vi "Benchmark Replace.vi"() -> ()   [LabVIEW 2017]
uses:
  Source/LookupTable/LookupTable.lvclass/LookupTable.ctl
  fb17a209-de8c-4f41-abf7-ab837125ba6b.vi
  bfc32706-22d1-41c7-b150-1593975a2be3.vi
  Source/LookupTable/Read Table Reference.vi
  Source/LookupTable/LookupTable.lvclass
panel:
  in  "Numeric":i32=100000
  out "Waveform Chart":cluster{dbl, dbl, dbl}(graph)
  out "Variant DVR":dbl
  out "Variant by value":dbl
  out "Composed Lookup Table":dbl
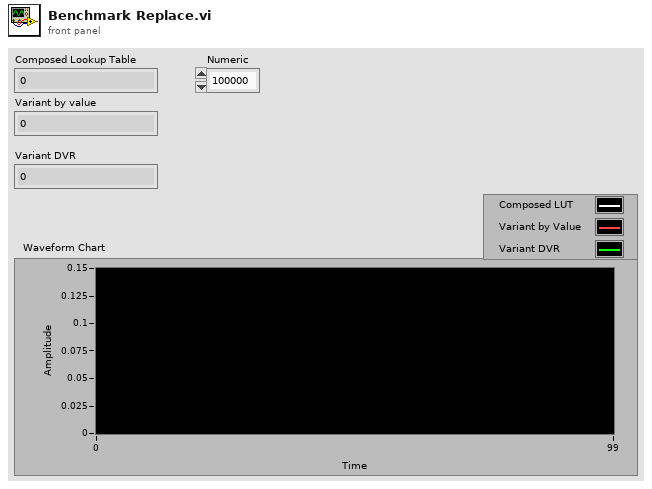
[diagram p1: front panel]
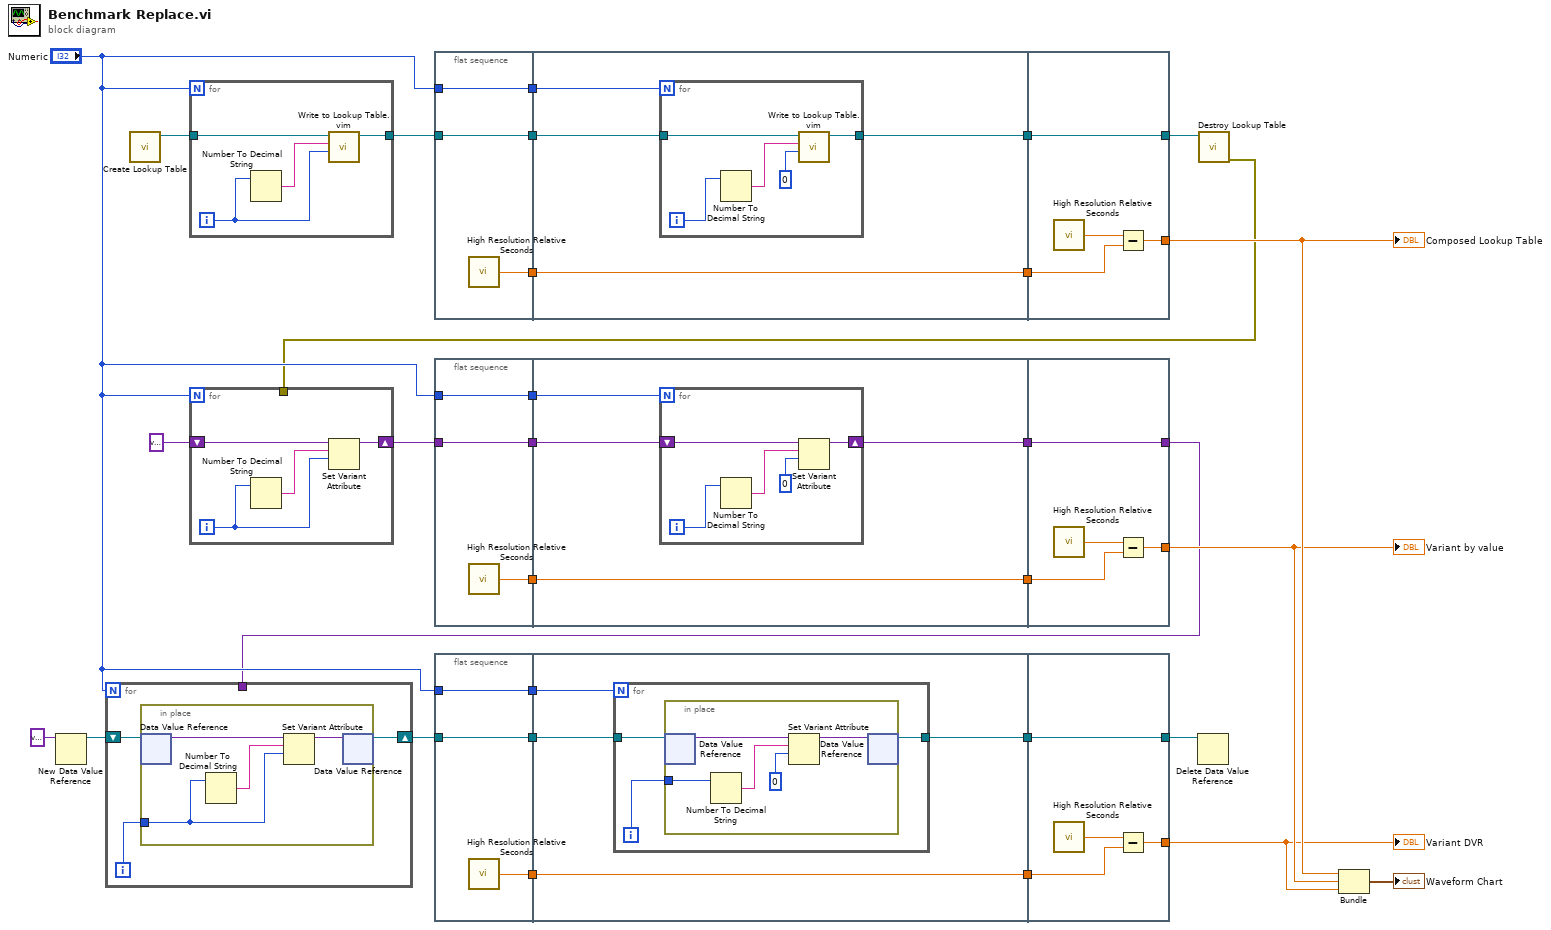
[diagram p0: block diagram]
diagram:
  n1 = New Data Value Reference(data value=variant) -> (data value reference=w11:refnum<data-value>)  [unwired: 1 in, 1 out]
  n2 = for {
    N: "Numeric" -> [_]
    shift-right: [w33] -> w10
    shift-left: w11 -> [w34]
    tunnel: w2 -> [_]
    i -> [w32]
    n3 = in-place {
      in-place-border: w32 -> [w35]
      n4 = in-place-dvr #1(w34) -> (w37:variant)  [unwired: 1 out]
      n5 = Number To Decimal String(number=w35) -> (decimal integer string=w38:string)  [unwired: 1 in]
      n6 = Set Variant Attribute(Variant=w37, name=w38, value=w35) -> (Variant out=w36:variant)  [unwired: 1 in, 2 out]
      n7 = in-place-dvr #1(w36) -> (w33:refnum<data-value>)  [unwired: 1 out]
    }
  }
  n8 = call "Create Lookup Table.vi"() -> ("LookupTable Reference"=w26:refnum<data-value>)  [unwired: 10 in, 1 out]
  n9 = for {
    N: "Numeric" -> [_]
    tunnel: [w40] -> w24
    tunnel: w26 -> [w39]
    i -> [w41]
    n10 = Number To Decimal String(number=w41) -> (decimal integer string=w42:string)  [unwired: 1 in]
    n11 = call "Write to Lookup Table.vim"("Item"=w41, "Item Name"=w42, "LookupTable Reference"=w39) -> ("LookupTable Reference Out"=w40:refnum<data-value>)  [unwired: 6 in, 2 out]
  }
  n12 = flat-sequence {
    tunnel: [w45] -> w31
    tunnel: [w44] -> w25
    tunnel: w24 -> [w44]
    tunnel: [w43] -> w19
    tunnel: "Numeric" -> [w43]
    tunnel: w31 -> [w49]
    tunnel: [w49] -> w30
    tunnel: w25 -> [w48]
    tunnel: [w47] -> w22
    tunnel: w19 -> [w46]
    tunnel: w30 -> [w57]
    tunnel: [w56] -> w7
    tunnel: [w55] -> w23
    tunnel: w22 -> [w55]
    frame #0 {
      n13 = call <vilib>:"High Resolution Relative Seconds.vi"() -> ("relative seconds"=w45:dbl)
    }
    frame #1 {
      n14 = for {
        N: w46 -> [_]
        tunnel: [w52] -> w47
        tunnel: w48 -> [w51]
        i -> [w53]
        n15 = Number To Decimal String(number=w53) -> (decimal integer string=w54:string)  [unwired: 1 in]
        n16 = call "Write to Lookup Table.vim"("Item"=0, "Item Name"=w54, "LookupTable Reference"=w51) -> ("LookupTable Reference Out"=w52:refnum<data-value>)  [unwired: 6 in, 2 out]
      }
    }
    frame #2 {
      n17 = call <vilib>:"High Resolution Relative Seconds.vi"() -> ("relative seconds"=w58:dbl)
      n18 = Subtract(x=w58, y=w57) -> (x-y=w56:dbl)
    }
  }
  n19 = flat-sequence {
    tunnel: [w61] -> w29
    tunnel: [w60] -> w21
    tunnel: w20 -> [w60]
    tunnel: "Numeric" -> [w59]
    tunnel: [w59] -> w18
    tunnel: w29 -> [w65]
    tunnel: [w65] -> w28
    tunnel: w21 -> [w64]
    tunnel: w18 -> [w63]
    tunnel: [w62] -> w1
    tunnel: w28 -> [w73]
    tunnel: [w72] -> w6
    tunnel: [w71] -> w2
    tunnel: w1 -> [w71]
    frame #0 {
      n20 = call <vilib>:"High Resolution Relative Seconds.vi"() -> ("relative seconds"=w61:dbl)
    }
    frame #1 {
      n21 = for {
        N: w63 -> [_]
        shift-right: [w70] -> w62
        shift-left: w64 -> [w67]
        i -> [w68]
        n22 = Number To Decimal String(number=w68) -> (decimal integer string=w69:string)  [unwired: 1 in]
        n23 = Set Variant Attribute(Variant=w67, name=w69, value=0) -> (Variant out=w70:variant)  [unwired: 1 in, 2 out]
      }
    }
    frame #2 {
      n24 = call <vilib>:"High Resolution Relative Seconds.vi"() -> ("relative seconds"=w74:dbl)
      n25 = Subtract(x=w74, y=w73) -> (x-y=w72:dbl)
    }
  }
  n26 = flat-sequence {
    tunnel: [w77] -> w17
    tunnel: [w76] -> w16
    tunnel: w10 -> [w76]
    tunnel: "Numeric" -> [w75]
    tunnel: [w75] -> w15
    tunnel: w17 -> [w81]
    tunnel: [w81] -> w14
    tunnel: w16 -> [w80]
    tunnel: w15 -> [w78]
    tunnel: [w79] -> w13
    tunnel: w14 -> [w92]
    tunnel: [w91] -> w5
    tunnel: [w90] -> w9
    tunnel: w13 -> [w90]
    frame #0 {
      n27 = call <vilib>:"High Resolution Relative Seconds.vi"() -> ("relative seconds"=w77:dbl)
    }
    frame #1 {
      n28 = for {
        N: w78 -> [_]
        tunnel: [w83] -> w79
        tunnel: w80 -> [w82]
        i -> [w84]
        n29 = in-place {
          in-place-border: w84 -> [w88]
          n30 = in-place-dvr #2(w82) -> (w87:variant)  [unwired: 1 out]
          n31 = Number To Decimal String(number=w88) -> (decimal integer string=w89:string)  [unwired: 1 in]
          n32 = Set Variant Attribute(Variant=w87, name=w89, value=0) -> (Variant out=w86:variant)  [unwired: 1 in, 2 out]
          n33 = in-place-dvr #2(w86) -> (w83:refnum<data-value>)  [unwired: 1 out]
        }
      }
    }
    frame #2 {
      n34 = call <vilib>:"High Resolution Relative Seconds.vi"() -> ("relative seconds"=w93:dbl)
      n35 = Subtract(x=w93, y=w92) -> (x-y=w91:dbl)
    }
  }
  n36 = Delete Data Value Reference(data value reference=w9) -> ()  [unwired: 1 in, 2 out]
  n37 = call "Destroy Lookup Table.vi"("LookupTable Reference"=w23) -> ("error out"=w3:errorcluster)  [unwired: 10 in]
  n38 = for {
    N: "Numeric" -> [_]
    shift-right: [w97] -> w20
    shift-left: variant -> [w94]
    tunnel: w3 -> [_]
    i -> [w95]
    n39 = Number To Decimal String(number=w95) -> (decimal integer string=w96:string)  [unwired: 1 in]
    n40 = Set Variant Attribute(Variant=w94, name=w96, value=w95) -> (Variant out=w97:variant)  [unwired: 1 in, 2 out]
  }
  n41 = Bundle(w7, w6, w5) -> (→"Waveform Chart":cluster{dbl, dbl, dbl})  [unwired: 1 in]
  "Composed Lookup Table" <- w7
  "Variant by value" <- w6
  "Variant DVR" <- w5
